vi "pulse from memory 8spc_v3.vi"(9 "referenses":T3={"clock x2"="IO Socket\\Data Clock 2x", "Memory In"="pulse on memory"}, 10 "start this pulse":bool, 11 "PDW":T1={"PW"=0, "frequency shift"=0.0, "amp"=0.9999923706054688, "mode type"=enum."CW", "mode depth"=0, "mode filter"=0, "phase shift"=0.0, "pulse shape filter"=0} {"frequency shift" format="%#_12f"}) -> (1 "free DDS":bool, 3 "IQ_out":T4[](array[typedef]))   [LabVIEW 2021]
uses:
  <instrlib>/_niInstr/DSP/v1/Shared/Public/IQ Data.ctl
  pulse_tx_vis/pdw.ctl
  pulse_tx_vis/CTL/mode_type.ctl
  <instrlib>/_niInstr/DSP/v1/FPGA/Public/Sub VIs/Data Conversion/U32 to IQ - 1 spc - S18.1.vi
  <instrlib>/FlexRIO/API/UsrFpgaDsp/v1/FPGA/HbInt/UsrFpgaDspHbIntIQ_8Cps_1xOC_BWper2_96dB.vi
  <instrlib>/FlexRIO/API/UsrFpgaDsp/v1/FPGA/HbInt/UsrFpgaDspHbIntIQ_4Cps_1xOC_BWper2_89dB.vi
  <instrlib>/FlexRIO/API/UsrFpgaDsp/v1/FPGA/HbInt/UsrFpgaDspHbIntIQ_2Cps_1xOC_BWper2_89dB.vi
  <vilib>/rvi/DataTransferAndStorage/Container/Common/niFpgaContainerExecOnDevCompGetState.vi
  <vilib>/rvi/Emulation/niFpgaEmulationIsFPGAContextNoSignature.vi
  <vilib>/rvi/DataTransferAndStorage/Container/Common/niFpgaContainerGetUniqueNameForEmu.vi
  <vilib>/rvi/Emulation/niFpgaProcessEmulError.vi
  <vilib>/rvi/Emulation/niFpgaSctlEmulationGetInTimedLoop.vi
  <vilib>/rvi/errors/nirviReportUnexpectedCaseInternalError (U32).vi
  <vilib>/rvi/Memory/Memory_Emulation/niFpgaMemoryEmulationCacheClearOnFirstRun.vi
  <vilib>/rvi/Memory/Memory_Emulation/nirvimemoryEmulationManagerCache_MakeExclusive.vi
  <vilib>/rvi/Memory/Memory_Emulation/niFpgaMemoryEmulationValidateCache.vi
  <vilib>/rvi/Memory/Memory_Emulation/nirvimemoryEmulationManagerCache_InsertValue.vi
  <vilib>/Utility/error.llb/Clear Errors.vi
  <vilib>/rvi/Memory/Memory_Emulation/nirvimemoryEmulationManagerCache_ReleaseExclusive.vi
  <vilib>/rvi/Memory/Memory_Emulation/nirvimemoryEmulationManagerCache_GetValue.vi
  <vilib>/rvi/Memory/Memory_Emulation/nirvimemoryEmulationManagerCache_SetValue.vi
  <vilib>/rvi/Emulation/niFpgaSctlEmulationResourceMgr.vi
  <instrlib>/FlexRIO/API/UsrFpgaDsp/v1/FPGA/HbInt/UsrFpgaDspHbIntIQ_1Spc_2xOC_BWper2_89dB.vi
  <instrlib>/FlexRIO/API/UsrFpgaDsp/v1/FPGA/HbInt/UsrFpgaDspHbIntIQ_2Spc_2xOC_BWper2_89dB.vi
  <instrlib>/FlexRIO/API/UsrFpgaDsp/v1/FPGA/HbInt/UsrFpgaDspHbIntIQ_4Spc_2xOC_BWper2_89dB.vi
  <instrlib>/_niInstr/DSP/v1/FPGA/Public/Sub VIs/Frequency Shift/Frequency Shift - 8 spc.vi
  <instrlib>/_niInstr/Basic Elements/v1/FPGA/Private/Count Up U32.vi
  <instrlib>/_niInstr/Basic Elements/v1/FPGA/Private/Count Up U16.vi
  <vilib>/rvi/DataTransferAndStorage/Container/XNode/niFpgaContainer.xnode
  <vilib>/rvi/Memory/Memory_Emulation/niFpgaMemoryEmulationRefIn.vi
  <instrlib>/_niInstr/DSP/v1/Shared/niInstr DSP v1 Shared.lvlib
  <instrlib>/_niInstr/DSP/v1/FPGA/niInstr DSP v1 FPGA.lvlib
  <instrlib>/_niInstr/Basic Elements/v1/FPGA/niInstr Basic Elements v1 FPGA.lvlib
  <instrlib>/FlexRIO/API/UsrFpgaDsp/v1/FPGA/HbInt/UsrFpgaDsp HbInt v1 FPGA.lvlib
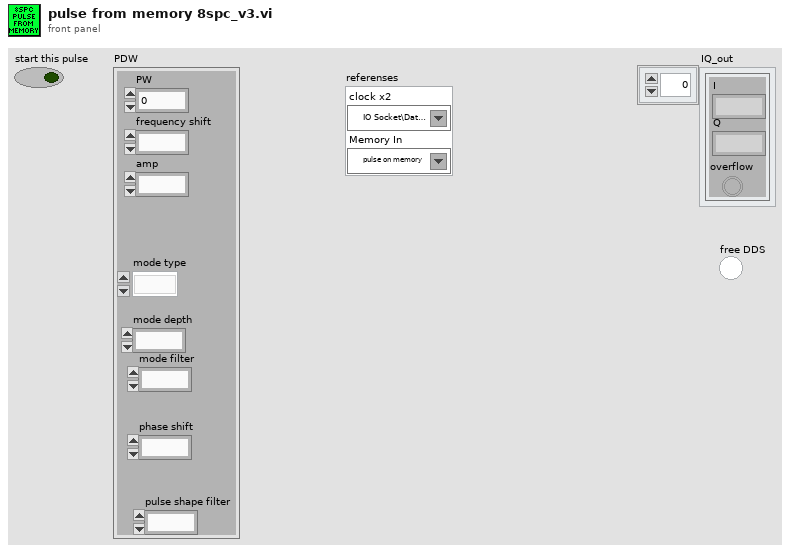
[diagram p1: front panel]
types:
  T1 = typedef "pdw.ctl" = cluster{"PW":u32, "frequency shift":fxp<+/-,48,0>, "amp":fxp<+/-,18,1>, "mode type":T2, "mode depth":u32, "mode filter":u8, "phase shift":fxp<+/-,16,1>, "pulse shape filter":u8}
  T2 = typedef "mode_type.ctl" = enum8{"CW", "from memory 1", "NC - cw", "LFM", "BPSK", "QPSK"}
  T3 = cluster{"clock x2":refnum<k21>, "Memory In":refnum<k21>}
  T4 = typedef "niInstr DSP v1 Shared.lvlib/IQ Data.ctl" = cluster{"I":fxp<+/-,18,1>, "Q":fxp<+/-,18,1>, "overflow":bool}
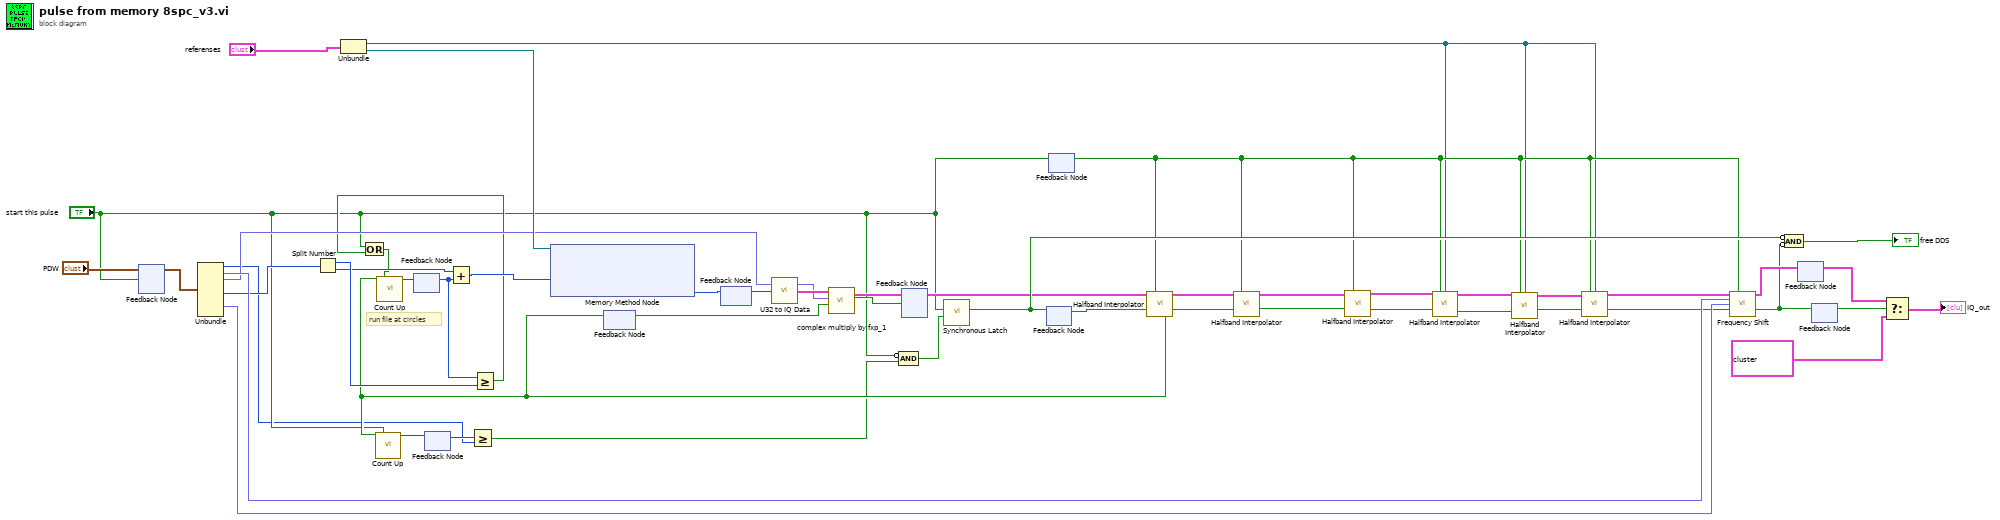
[diagram p0: block diagram]
diagram:
  # "run file at circles"
  n1 = feedback #1() -> (w42:T1)  [unwired: 1 in]
  n2 = feedback-in #1("PDW", "start this pulse") -> ()
  n3 = Unbundle(w42) -> ("PW"=w2:u32, "frequency shift"=w48:fxp<+/-,48,0>, "amp"=w36:fxp<+/-,18,1>, "mode depth"=w9:u32, "phase shift"=w47:fxp<+/-,16,1>)  [unwired: 3 out]
  n4 = Split Number(x=w9) -> (hi(x)=w41:u16, lo(x)=w35:u16)
  n5 = Unbundle("referenses") -> ("clock x2"=w10:refnum<k21>, "Memory In"=w44:refnum<k21>)
  n6 = feedback #2() -> (w33:u16)  [unwired: 1 in]
  n7 = feedback #3() -> (w3:u32)  [unwired: 1 in]
  n8 = Add(x=w35, y=w33) -> (x+y=w32:u16)
  n9 = Greater Or Equal?(x=w3, y=w2) -> (x >= y?=w1:bool)
  n10 = Greater Or Equal?(x=w33, y=w41) -> (x >= y?=w6:bool)
  n11 = Or(x="start this pulse", y=w6) -> (x .or. y?=w7:bool)
  n12 = xnode ("Memory Method Node")("Address"=w32, "Memory In"=w44) -> ("Data"=w52:u32)  [unwired: 1 out]
  n13 = feedback #4() -> (w37:bool)  [unwired: 1 in]
  n14 = feedback #5() -> (w51:u32)  [unwired: 1 in]
  n15 = feedback-in #5(w52) -> ()
  n16 = call-poly <instrlib>:"U32 to IQ Data.vi"("U32 data"=w51) -> ("IQ data"=w39:T4)  [unwired: 14 in]
  n17 = call "complex multiply by fxp_1.vi"("input valid"=w37, "amp"=w36, "IQ data"=w39) -> ("data valid"=w40:bool, "output cluster"=w38:T4)  [unwired: 7 in]
  n18 = Compound Arithmetic op=AND(invert "start this pulse", w1) -> (w50:bool)
  n19 = feedback #6() -> (w15:T4)  [unwired: 1 in]
  n20 = feedback-in #6(w38, w40) -> ()
  n21 = call <instrlib>:"Synchronous Latch.vi"("clear"=w50, "set"="start this pulse") -> ("out"=w26:bool)  [unwired: 9 in]
  n22 = feedback #7() -> (w14:bool)  [unwired: 1 in]
  n23 = feedback-in #7(w26) -> ()
  n24 = feedback-in #8("start this pulse") -> ()
  n25 = feedback #8() -> (w11:bool)  [unwired: 1 in]
  n26 = call-poly "Halfband Interpolator.vi"("data in"=w15, "reset"=w11, "input valid"=w14) -> ("data out"=w25:T4, "output valid"=w16:bool, "ready for input"=w5:bool)  [unwired: 10 in]
  n27 = call-poly <instrlib>:"Count Up.vi"("increment"=w5, "reset"="start this pulse") -> ("count out"=w8:u32)  [unwired: 13 in]
  n28 = call-poly <instrlib>:"Count Up.vi"("increment"=w5, "reset"=w7) -> ("count out"=w34:u16)  [unwired: 13 in]
  n29 = feedback-in #2(w34) -> ()
  n30 = feedback-in #3(w8) -> ()
  n31 = feedback-in #4(w5) -> ()
  n32 = call-poly "Halfband Interpolator.vi"("data in"=w25, "reset"=w11, "input valid"=w16) -> ("data out"=w24:T4, "output valid"=w17:bool)  [unwired: 10 in, 1 out]
  n33 = call-poly "Halfband Interpolator.vi"("data in"=w24, "reset"=w11, "input valid"=w17) -> ("data out"=w23:T4, "output valid"=w18:bool)  [unwired: 10 in, 1 out]
  n34 = call-poly "Halfband Interpolator.vi"("data in"=w23, "reset"=w11, "clk2x"=w10, "input valid"=w18) -> ("data out"=w22:T4[], "output valid"=w19:bool)  [unwired: 9 in, 1 out]
  n35 = call-poly "Halfband Interpolator.vi"("data in"=w22, "reset"=w11, "clk2x"=w10, "input valid"=w19) -> ("data out"=w21:T4[], "output valid"=w20:bool)  [unwired: 9 in, 1 out]
  n36 = call-poly "Halfband Interpolator.vi"("data in"=w21, "reset"=w11, "clk2x"=w10, "input valid"=w20) -> ("data out"=w12:T4[], "output valid"=w13:bool)  [unwired: 9 in, 1 out]
  n37 = call-poly <instrlib>:"Frequency Shift.vi"("data in"=w12, "reset"=w11, "frequency shift"=w48, "phase"=w47, "input valid"=w13) -> ("data out"=w31:T4[], "output valid"=w29:bool)  [unwired: 7 in, 2 out]
  n38 = Compound Arithmetic op=AND(invert w26, invert w29) -> (→"free DDS":bool)
  n39 = feedback #9() -> (w30:T4[])  [unwired: 1 in]
  n40 = feedback-in #9(w31) -> ()
  n41 = feedback #10() -> (w28:bool)  [unwired: 1 in]
  n42 = feedback-in #10(w29) -> ()
  n43 = Select(t=w30, s=w28, f=T4[] [{"I"=0.0, "Q"=0.0, "overflow"=FALSE}, {"I"=0.0, "Q"=0.0, "overflow"=FALSE}, {"I"=0.0, "Q"=0.0, "overflow"=FALSE}, {"I"=0.0, "Q"=0.0, "overflow"=FALSE}, {"I"=0.0, "Q"=0.0, "overflow"=FALSE}, {"I"=0.0, "Q"=0.0, "overflow"=FALSE}, {"I"=0.0, "Q"=0.0, "overflow"=FALSE}, {"I"=0.0, "Q"=0.0, "overflow"=FALSE}] ("data out")) -> (s? t:f=→"IQ_out":T4[])
